vi "Read Password.vi"(8 "error in (no error)":errorcluster, 11 "BaseMeasurement in":refnum<class "BaseMeasurement.lvclass">) -> (0 "error out":errorcluster, 2 "Password":string, 3 "BaseMeasurement out":refnum<class "BaseMeasurement.lvclass">)   [LabVIEW 2013, in "BaseMeasurement.lvclass"]
doc: "Reads the password used to access the data file."
uses:
  BaseMeasurement.lvclass
  BaseMeasurement.lvclass/BaseMeasurement.ctl
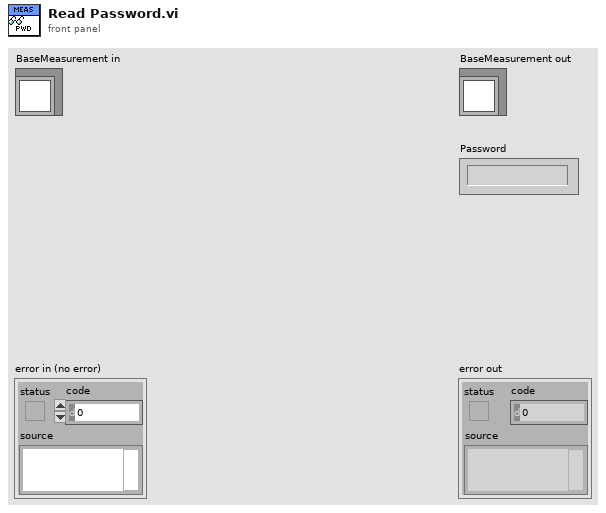
[diagram p1: front panel]
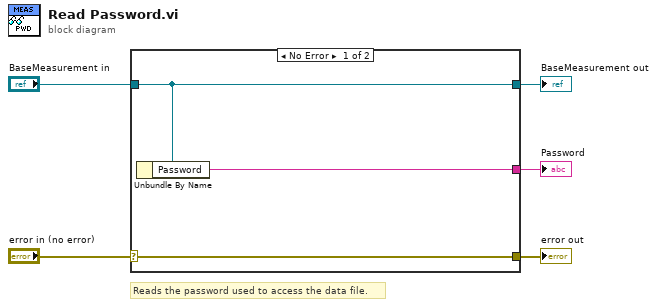
[diagram p0: block diagram]
diagram:
  # "Reads the password used to access the data file."
  n1 = case shown="No Error" "error in (no error)" {
    selector: "error in (no error)" -> [w8 w9]
    tunnel: [w8 w9] -> w4
    tunnel: [w7 w10] -> w2
    tunnel: "BaseMeasurement in" -> [w7 w10]
    tunnel: [w6 _] -> w1
    frame No Error {
      n2 = Unbundle By Name(w7) -> ("Password"=w6:string)
    }
    frame Error {
    }
  }
  "error out" <- w4
  "BaseMeasurement out" <- w2
  "Password" <- w1
